vi "motor paso a paso.vi"() -> ()   [LabVIEW 2016]
uses:
  <vilib>/LabVIEW Interface for Arduino/Type Defs/Board Type.ctl
  <vilib>/LabVIEW Interface for Arduino/Type Defs/Connection Type.ctl
  <vilib>/LabVIEW Interface for Arduino/LabVIEW Interface for Arduino.lvlib
panel:
  out "Steps remaining":u16
  out "Steps Remaining?":bool
  in  "Stop Button":bool
  in  "Velocidad":u32(slide) scale=0.0..100.0
  in  "Pasos":u32(knob) scale=0.0..1000.0
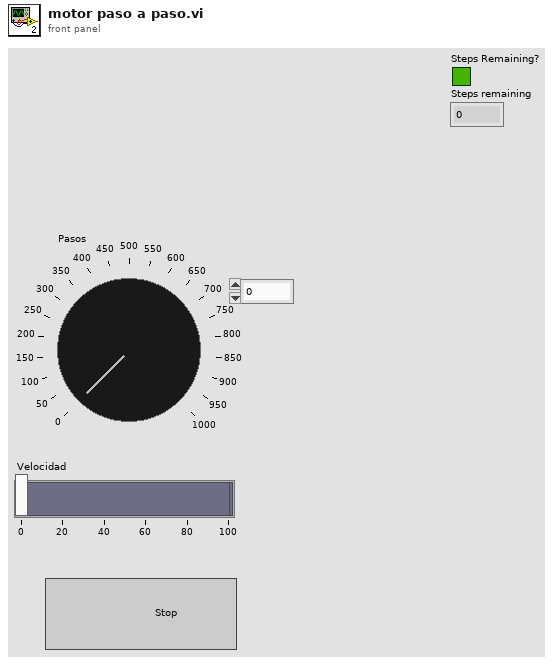
[diagram p1: front panel]
types:
  T1 = typedef "LabVIEW Interface for Arduino.lvlib/Connection Type.ctl" = enum8{"USB / Serial", "XBEE", "BlueSmirf (Bluetooth)"}
  T2 = typedef "LabVIEW Interface for Arduino.lvlib/Board Type.ctl" = enum16{"Uno", "Dimuelanove w/Atmega 328", "Mega 2560"}
  T3 = typedef "LabVIEW Interface for Arduino.lvlib/Arduino Resource.ctl" = cluster{"VISA resource":refnum<visa-resource-name>, "Board Type":T2, "Connection Type":enum8{"USB / Serial"}, "Bytes Per Packet (15)":u8}
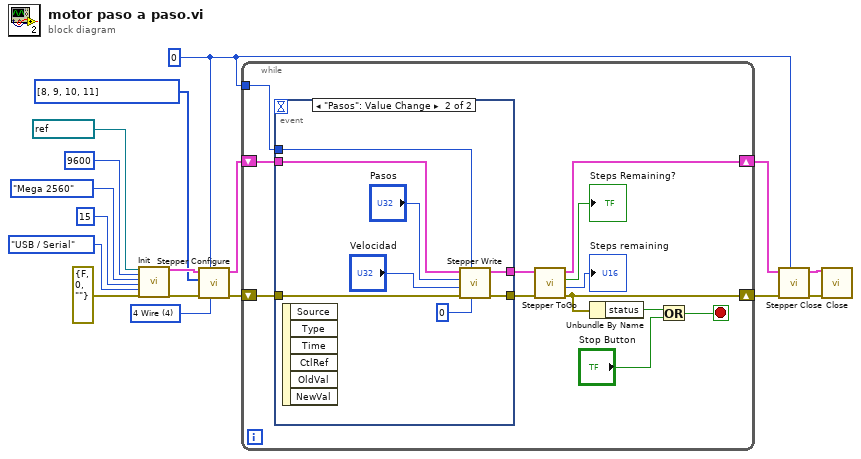
[diagram p0: block diagram]
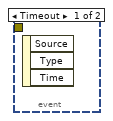
[diagram p2: hidden frame]
diagram:
  w9 = u8 4 items=["2 Wire (Pulse & Direction)"=1, "2 Wire"=2, "4 Wire"=4, "EasyDriver"=6, "AF Motor Shield (Stepper 1 & 2 Only)"=5] ("Control Method")
  w5 = u8 0 ("Stepper #")
  n1 = call <vilib>:"Init.vi"("VISA resource"=refnum<visa-resource-name> "COM6", "Baud Rate (115200)"=u32 9600, "Board Type (Uno)"=Board_Type."Mega 2560", "Bytes Per Packet (15)"=u32 15, "Connection Type (USB/Serial)"=Connection_Type."USB / Serial", "error in"=errorcluster {"status"=FALSE, "code"=0, "source"=""}) -> ("Arduino Resource"=w10:T3, "error out"=w11:errorcluster)  [unwired: 12 in]
  n2 = call <vilib>:"Stepper Configure.vi"("Control Method"=w9, "Stepper #"=w5, "error in"=w11, "Stepper Pins"=u8[] [8, 9, 10, 11], "Arduino Resource"=w10) -> ("error out"=w6:errorcluster, "Arduino Resource Out"=w7:T3)  [unwired: 5 in]
  n3 = while {
    shift-right: [w22] -> w4
    shift-left: w7 -> [w29]
    shift-right: [w18] -> w3
    shift-left: w6 -> [w28]
    tunnel: w5 -> [w27]
    stop <- w26 stop-if-true
    n4 = event shown="[1] \"Pasos\": Value Change" {
      selector: _ -> [_ _]
      dyn-events: _ -> [_ _]
      timeout: _ -> [_ _]
      tunnel: w29 -> [_ w37]
      tunnel: w28 -> [_ w36]
      tunnel: w27 -> [_ w33]
      tunnel: [_ w31] -> w23
      tunnel: [_ w30] -> w21
      event Timeout {
        n5 = event-data() -> ()  [unwired: 1 in, 3 out]
      }
      event "Pasos": Value Change {
        n6 = event-data() -> ()  [unwired: 1 in, 6 out]
        n7 = call <vilib>:"Stepper Write.vi"("Set Acceleration (0 to disable)"=i16 0, "Stepper #"=w33, "error in"=w36, "Set Speed (Steps per Second)"="Velocidad", "# of Steps to Move"="Pasos", "Arduino Resource"=w37) -> ("error out"=w30:errorcluster, "Arduino Resource Out"=w31:T3)  [unwired: 4 in]
      }
    }
    n8 = call <vilib>:"Stepper ToGo.vi"("error in"=w21, "Arduino Resource"=w23) -> ("error out"=w18:errorcluster, "Steps remaining"=→"Steps remaining":u16, "Steps Remaining?"=→"Steps Remaining?":bool, "Arduino Resource Out"=w22:T3)  [unwired: 6 in]
    n9 = Unbundle By Name(w18) -> ("status"=w24:bool)
    n10 = Or(x=w24, y="Stop Button") -> (x .or. y?=w26:bool)
  }
  n11 = call <vilib>:"Stepper Close.vi"("Stepper #"=w5, "error in"=w3, "Arduino Resource"=w4) -> ("error out"=w1:errorcluster, "Arduino Resource Out"=w2:T3)  [unwired: 7 in]
  n12 = call <vilib>:"Close.vi"("Arduino Resource"=w2, "error in"=w1) -> ()  [unwired: 13 in, 1 out]
